vi "setVerticalCoupling.vi"(7 "Chn":string, 8 "error in (no error)":errorcluster, 10 "Coupling":T1, 11 "ScopeNi in":refnum<class "ScopeNi.lvclass">) -> (0 "error out":errorcluster, 3 "ScopeNi out":refnum<class "ScopeNi.lvclass">)   [LabVIEW 2023, in "ScopeNi.lvclass"]
doc: "<b>Author:</b> Wolfgang\n<b>Description:</b> specify the input coupling of the channel."
uses:
  ScopeNi.lvclass
  Data/scopeChnCoupling.ctl
  ScopeNi.lvclass/ScopeNi.ctl
  sweScope.lvlib
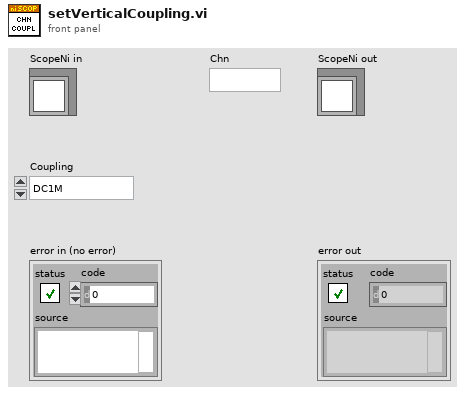
[diagram p1: front panel]
types:
  T1 = typedef "sweScope.lvlib/scopeChnCoupling.ctl" = enum16{"DC1M", "AC1M", "DC50", "GND"}
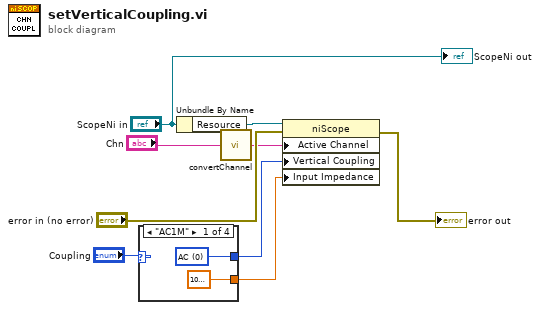
[diagram p0: block diagram]
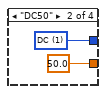
[diagram p2: hidden frame]
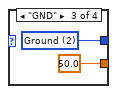
[diagram p3: hidden frame]
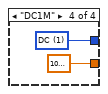
[diagram p4: hidden frame]
diagram:
  n1 = case shown="\"AC1M\"" "Coupling" {
    tunnel: [w11 w13 w15 w17] -> w4
    tunnel: [1000000.0 ("Vertical:Input Impedance") 50.0 ("Vertical:Input Impedance") 50.0 ("Vertical:Input Impedance") 1000000.0 ("Vertical:Input Impedance")] -> w2
    frame "AC1M" {
      w11 = 0 items=["AC", "DC", "Ground"] ("Vertical:Vertical Coupling")
    }
    frame "DC50" {
      w13 = 1 items=["AC", "DC", "Ground"] ("Vertical:Vertical Coupling")
    }
    frame "GND" {
      w15 = 2 items=["AC", "DC", "Ground"] ("Vertical:Vertical Coupling")
    }
    frame "DC1M" {
      w17 = 1 items=["AC", "DC", "Ground"] ("Vertical:Vertical Coupling")
    }
  }
  n2 = Unbundle By Name("ScopeNi in") -> ("Resource"=w9:refnum<k15>)
  n3 = call "convertChannel.vi"("Chn in"="Chn") -> ("Chn out"=w1:string)
  n4 = property class="niScope"(reference=w9, error in="error in (no error)", "Active Channel"=w1, "Vertical Coupling"=w4, "Input Impedance"=w2) -> (error out=→"error out":errorcluster)  [unwired: 1 out]
  "ScopeNi out" <- "ScopeNi in"
